vi "Send Message in Local Application.vi"(0 "message queue in":T3, 1 "receiver process (\"\" - local)":string, 5 "message":T1, 9 "timeout (-1 ms)":i32=-1, 11 "error in":errorcluster) -> (4 "message queue out":T3, 10 "timed out?":bool, 15 "error out":errorcluster)   [LabVIEW 2015, in "TLB` Template.lvlib" / "AMC.lvlib"]
doc: "This VI adds a message to the local message queue provided by the queue reference or to another message queue in the local application based on the receiver process name.TLB Prime - Application Template 1.3.0.24\nNorm Kirchner, NI Systems Engineering - NI\nCopyright (c) 2014, NI"
uses:
  AMC.lvlib
  Message Queue.ctl
  Message.ctl
  KeyedArray.ctl
  Generate Error.vi
  Tools_KeyedArray.lvlib
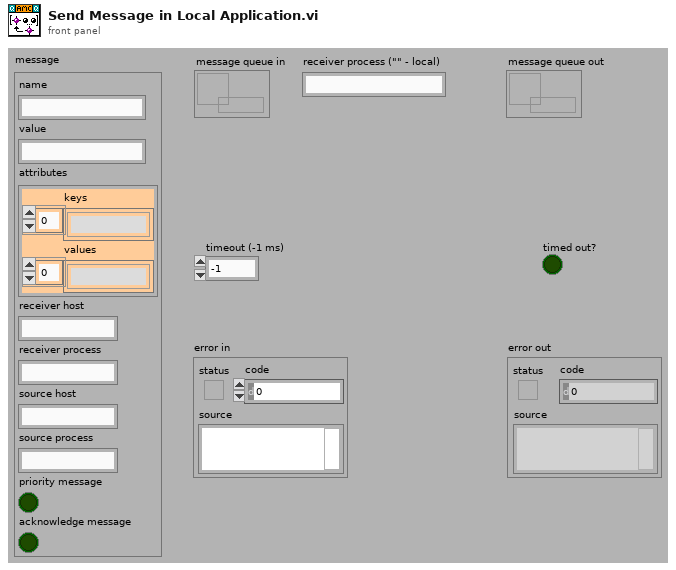
[diagram p1: front panel]
types:
  T1 = typedef "TLB` Template.lvlib/AMC.lvlib/Message.ctl" = cluster{"name":string, "value":string, "attributes":T2, "receiver host":string, "receiver process":string, "source host":string, "source process":string, "priority message":bool, "acknowledge message":bool}
  T2 = typedef "TLB` Template.lvlib/Tools_KeyedArray.lvlib/KeyedArray.ctl" = cluster{"keys":string[], "values":string[]}
  T3 = typedef "TLB` Template.lvlib/AMC.lvlib/Message Queue.ctl" = refnum<queue>
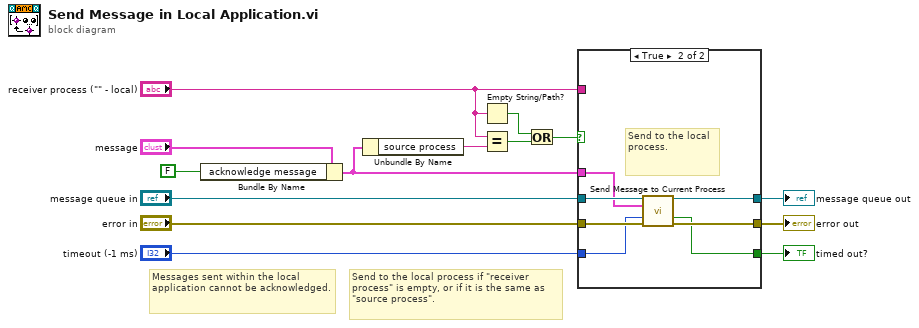
[diagram p0: block diagram]
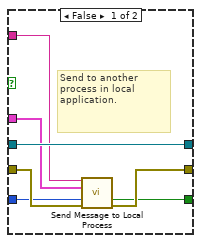
[diagram p2: hidden frame]
diagram:
  # "Send to the local process if \"receiver process\" is empty, or if it is the same as \"source process\"."
  # "Messages sent within the local application cannot be acknowledged."
  n1 = Bundle By Name(cluster="message", "acknowledge message"=FALSE) -> (w6:T1)
  n2 = Unbundle By Name(w6) -> ("source process"=w4:string)
  n3 = Empty String/Path?(string/path="receiver process (\"\" - local)") -> (empty?=w3:bool)
  n4 = Equal?(x="receiver process (\"\" - local)", y=w4) -> (x = y?=w2:bool)
  n5 = Or(x=w3, y=w2) -> (x .or. y?=w1:bool)
  n6 = case shown="True" w1 {
    tunnel: "message queue in" -> [w20 w28]
    tunnel: w6 -> [w18 w27]
    tunnel: "error in" -> [w21 w26]
    tunnel: [w20 w25] -> w12
    tunnel: [w19 w24] -> w11
    tunnel: "timeout (-1 ms)" -> [w17 w23]
    tunnel: [w16 w22] -> w9
    tunnel: "receiver process (\"\" - local)" -> [w15 _]
    frame False {
      # "Send to another process in local application."
      n7 = call "Send Message to Local Process.vi"("process name"=w15, "message"=w18, "timeout (-1 ms)"=w17, "error in"=w21) -> ("timed out?"=w16:bool, "error out"=w19:errorcluster)  [unwired: 10 in]
    }
    frame True {
      # "Send to the local process."
      n8 = call "Send Message to Current Process.vi"("message queue in"=w28, "message"=w27, "timeout (-1 ms)"=w23, "error in"=w26) -> ("message queue out"=w25:T3, "timed out?"=w22:bool, "error out"=w24:errorcluster)  [unwired: 9 in]
    }
  }
  "message queue out" <- w12
  "error out" <- w11
  "timed out?" <- w9
